vi "Data Displayer.vi"(6 "Fast Controls Only (F)":bool, 7 "Reset":bool, 8 "error in":errorcluster, 10 "All Data":T3 caption="All Data Cluster", 11 "Ref Data Array":T5) -> (0 "error out":errorcluster)   [LabVIEW 2018]
uses:
  Shared Controls/UI Ref Arrays.ctl
  Shared Controls/All Data Cluster.ctl
  Shared Controls/Acq Data.ctl
  Shared Controls/Calculated Data.ctl
  Shared Controls/Post-Analysis Data.ctl
  Gets APU Column Index.vi
panel:
  in  "Post-Analysis Data":T1
  in  "Calculated Values":T2
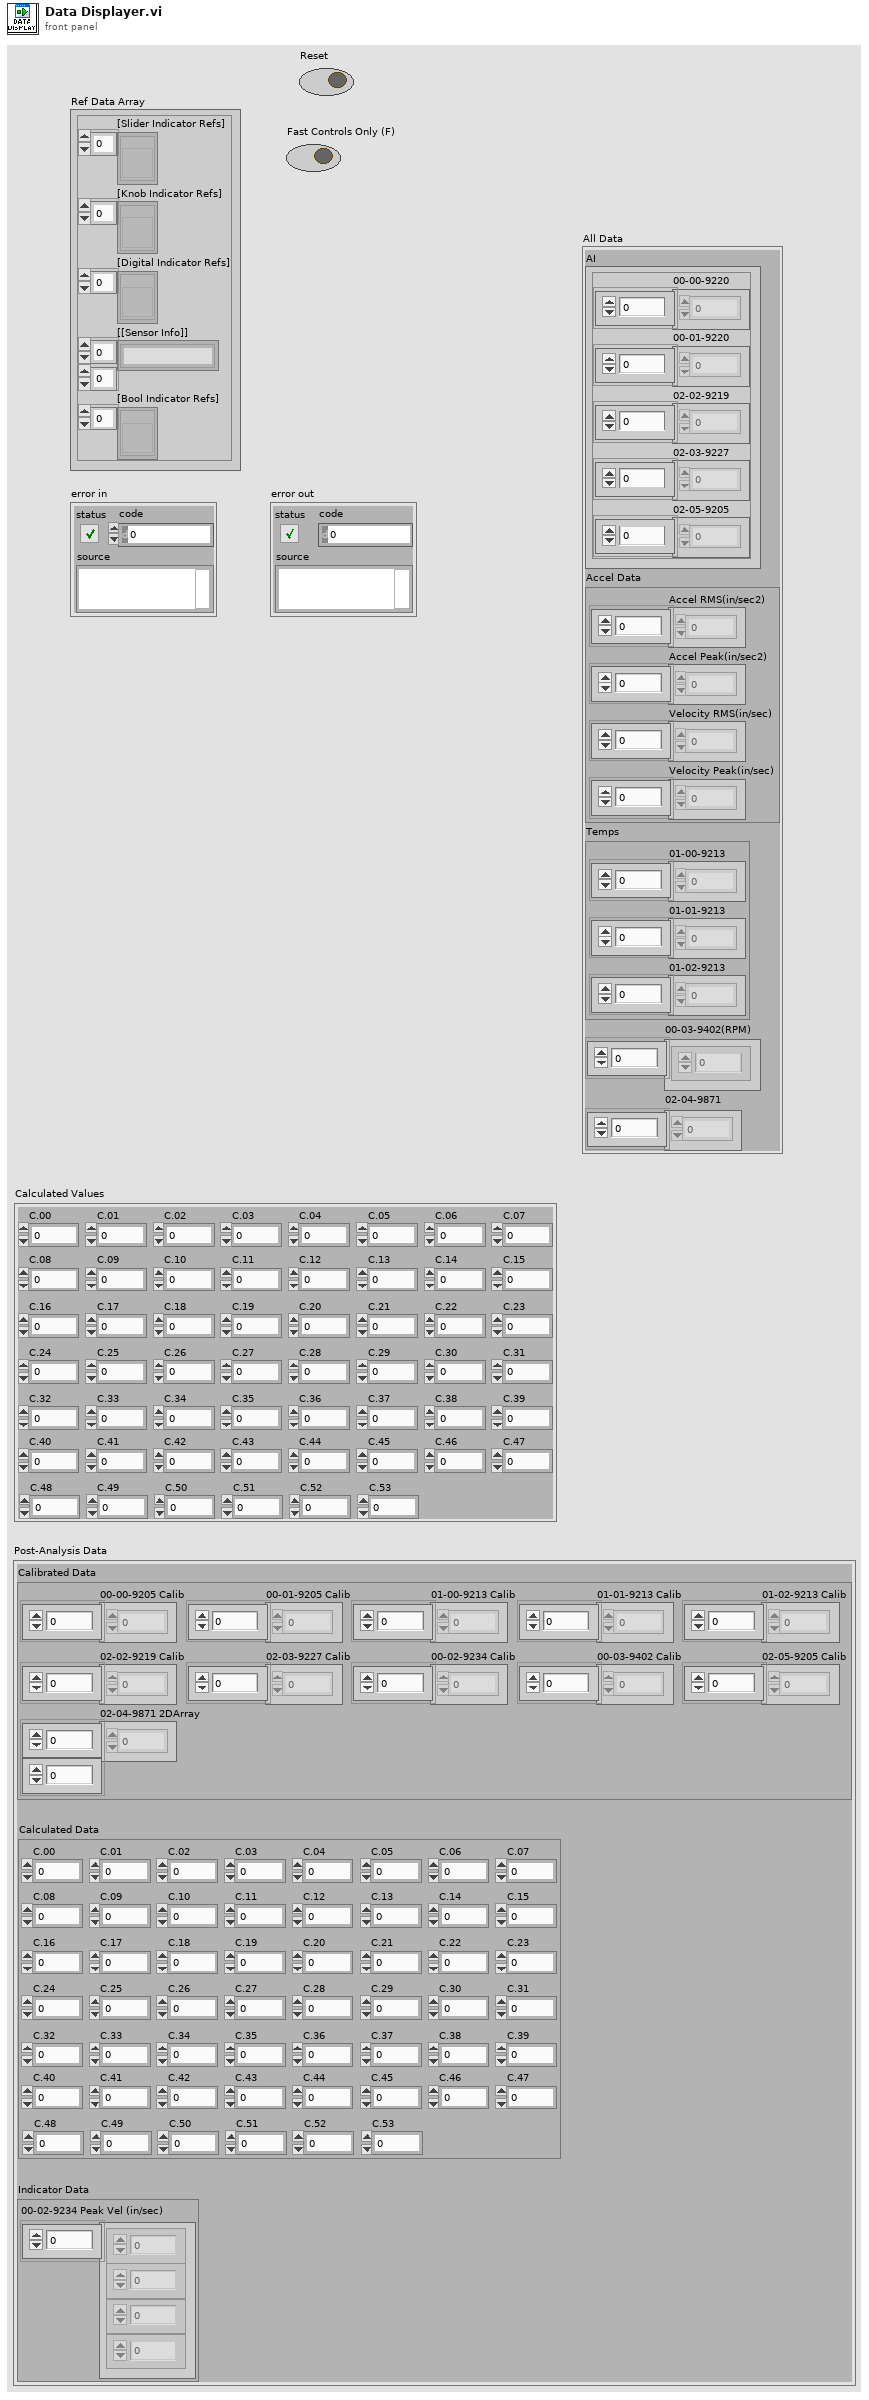
[diagram p1: front panel]
types:
  T1 = typedef "Post-Analysis Data.ctl" = cluster{"Calibrated Data":cluster{"00-00-9205 Calib":dbl[], "00-01-9205 Calib":dbl[], "01-00-9213 Calib":dbl[], "01-01-9213 Calib":dbl[], "01-02-9213 Calib":dbl[], "02-02-9219 Calib":dbl[], "02-03-9227 Calib":dbl[], "00-02-9234 Calib":dbl[], "00-03-9402 Calib":dbl[], "02-05-9205 Calib":dbl[], "02-04-9871 2DArray":dbl[][]}, "Calculated Data":T2, "Indicator Data":cluster{"00-02-9234 Peak Vel (in/sec)":dbl[]}}
  T2 = typedef "Calculated Data.ctl" = cluster{"C.00":dbl, "C.01":dbl, "C.02":dbl, "C.03":dbl, "C.04":dbl, "C.05":dbl, "C.06":dbl, "C.07":dbl, "C.08":dbl, "C.09":dbl, "C.10":dbl, "C.11":dbl, "C.12":dbl, "C.13":dbl, "C.14":dbl, "C.15":dbl, "C.16":dbl, "C.17":dbl, "C.18":dbl, "C.19":dbl, "C.20":dbl, "C.21":dbl, "C.22":dbl, "C.23":dbl, "C.24":dbl, "C.25":dbl, "C.26":dbl, "C.27":dbl, "C.28":dbl, "C.29":dbl, "C.30":dbl, "C.31":dbl, "C.32":dbl, "C.33":dbl, "C.34":dbl, "C.35":dbl, "C.36":dbl, "C.37":dbl, "C.38":dbl, "C.39":dbl, "C.40":dbl, "C.41":dbl, "C.42":dbl, "C.43":dbl, "C.44":dbl, "C.45":dbl, "C.46":dbl, "C.47":dbl, "C.48":dbl, "C.49":dbl, "C.50":dbl, "C.51":dbl, "C.52":dbl, "C.53":dbl}
  T3 = typedef "All Data Cluster.ctl" = cluster{"AI":T4, "Accel Data":cluster{"Accel RMS(in/sec2)":dbl[], "Accel Peak(in/sec2)":dbl[], "Velocity RMS(in/sec)":dbl[], "Velocity Peak(in/sec)":dbl[]}, "Temps":cluster{"01-00-9213":dbl[], "01-01-9213":dbl[], "01-02-9213":dbl[]}, "00-03-9402(RPM)":dbl[], "02-04-9871":dbl[]}
  T4 = typedef "Acq Data.ctl" = cluster{"00-00-9220":dbl[], "00-01-9220":dbl[], "02-02-9219":dbl[], "02-03-9227":dbl[], "02-05-9205":dbl[]}
  T5 = typedef "UI Ref Arrays.ctl" = cluster{"[Slider Indicator Refs]":refnum<vi>[], "[Knob Indicator Refs]":refnum<vi>[], "[Digital Indicator Refs]":refnum<vi>[], "[[Sensor Info]]":string[][], "[Bool Indicator Refs]":refnum<vi>[]}
  T6 = cluster{"Thresold Array":dbl[], "Label Text":string, "Ref type":enum16{"Not Found", "Knob", "Numeric", "Slide", "String", "Boolean"}, "BG Color":u32}
  T7 = typedef "Parsed Tag Cluster.ctl" = cluster{"Whole Tag":string, "# of Sections":u8, "Chassis":u8, "Slot":u8, "Module":string, "Channel":u8, "SubChannel":u8}
  T8 = cluster{"Thresold Array":dbl[], "Label Text":string, "Ref type":enum16{"Not Found", "Knob", "Numeric", "Slide", "String", "Boolean"}, "BG Color":u32}[]
  T9 = enum16{"Not Found", "Knob", "Numeric", "Slide", "String", "Boolean"}
  T10 = cluster{"Thresold Array":dbl[], "Label.Text":string, "Ref type":enum16{"Not Found", "Knob", "Numeric", "Slide", "String", "Boolean"}, "BG Color":u32}
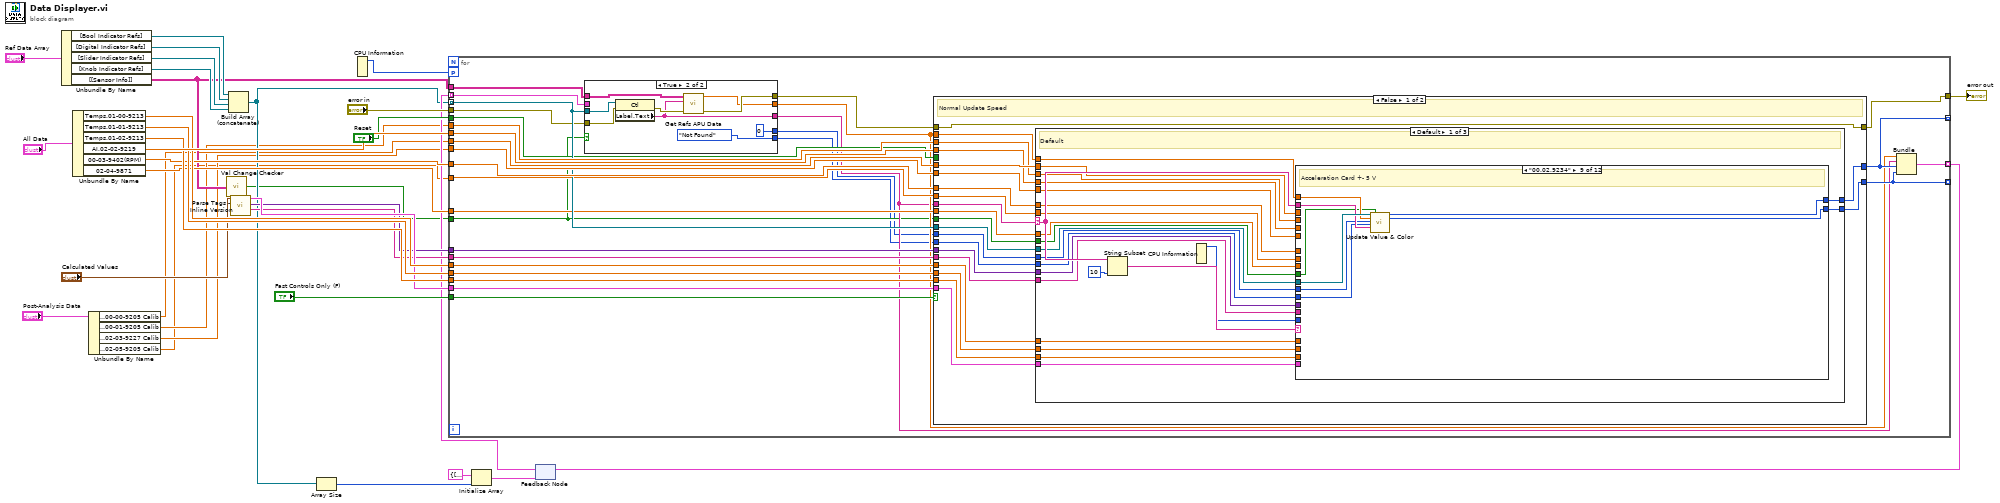
[diagram p0: block diagram]
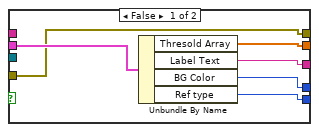
[diagram p2: hidden frame]
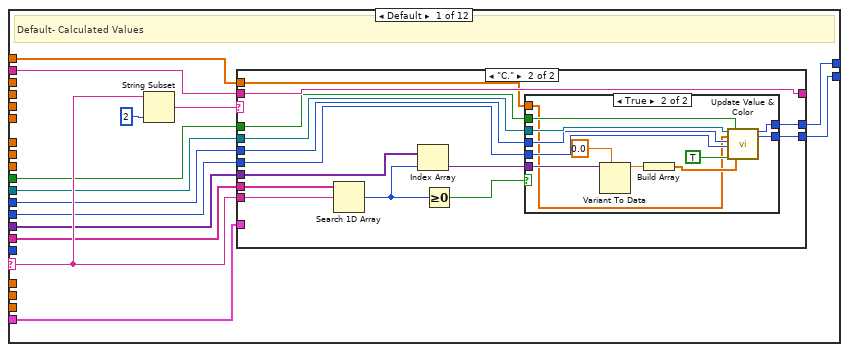
[diagram p3: hidden frame]
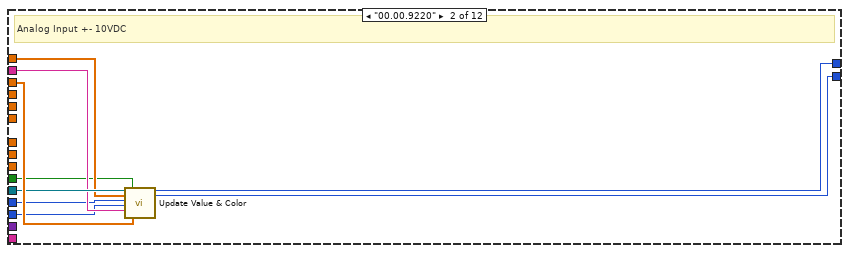
[diagram p6: hidden frame]
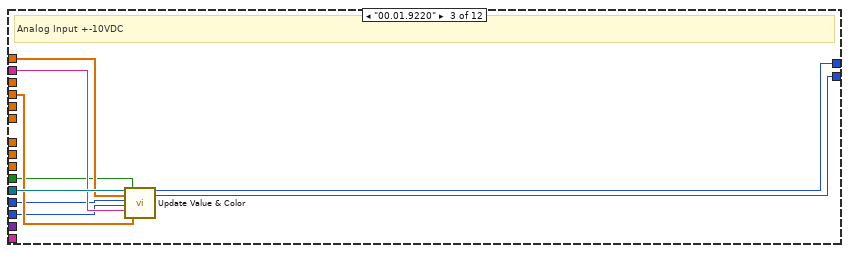
[diagram p7: hidden frame]
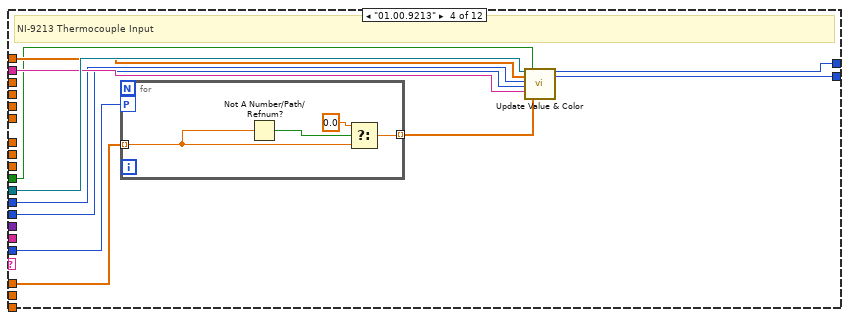
[diagram p8: hidden frame]
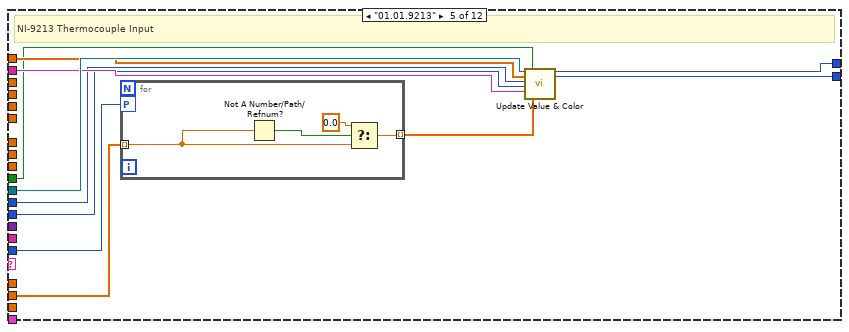
[diagram p9: hidden frame]
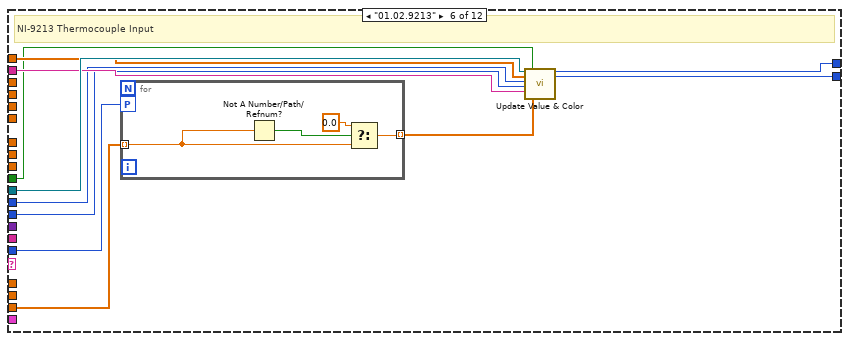
[diagram p10: hidden frame]
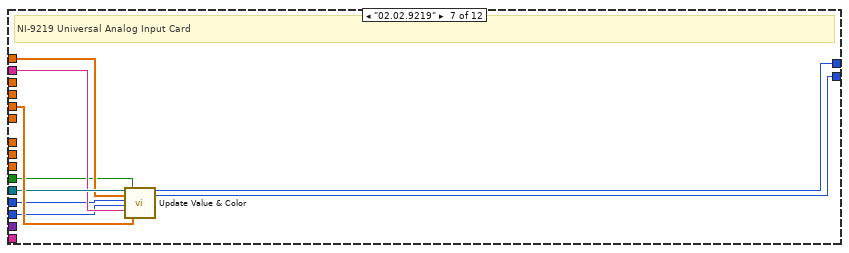
[diagram p11: hidden frame]
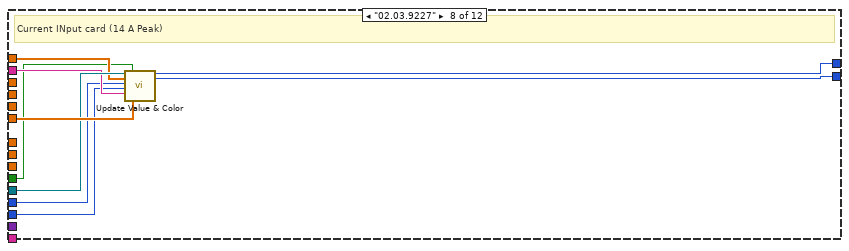
[diagram p12: hidden frame]
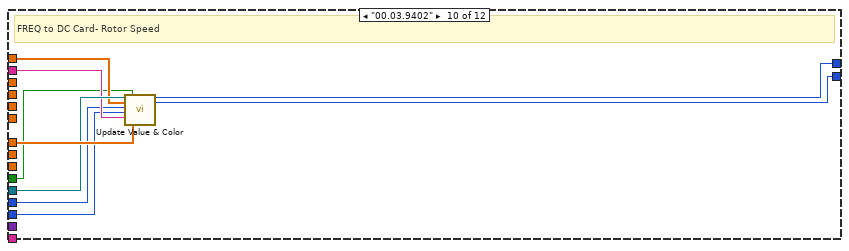
[diagram p13: hidden frame]
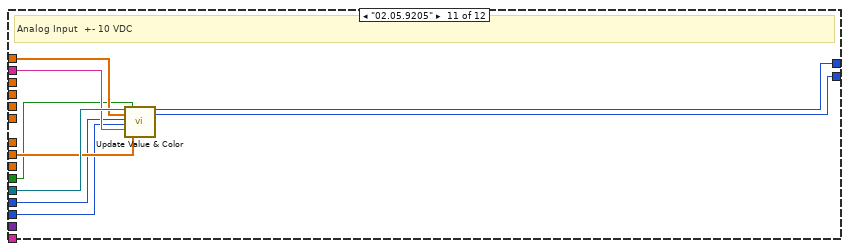
[diagram p14: hidden frame]
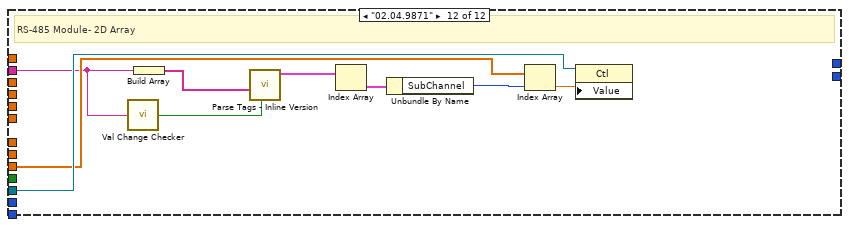
[diagram p15: hidden frame]
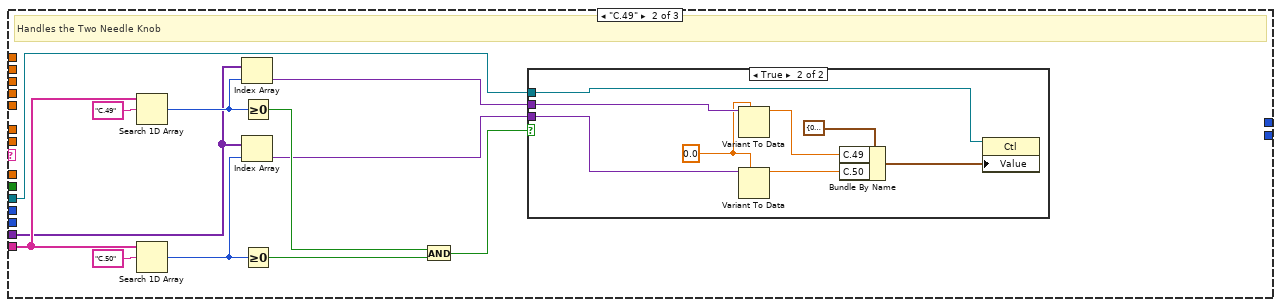
[diagram p16: hidden frame]
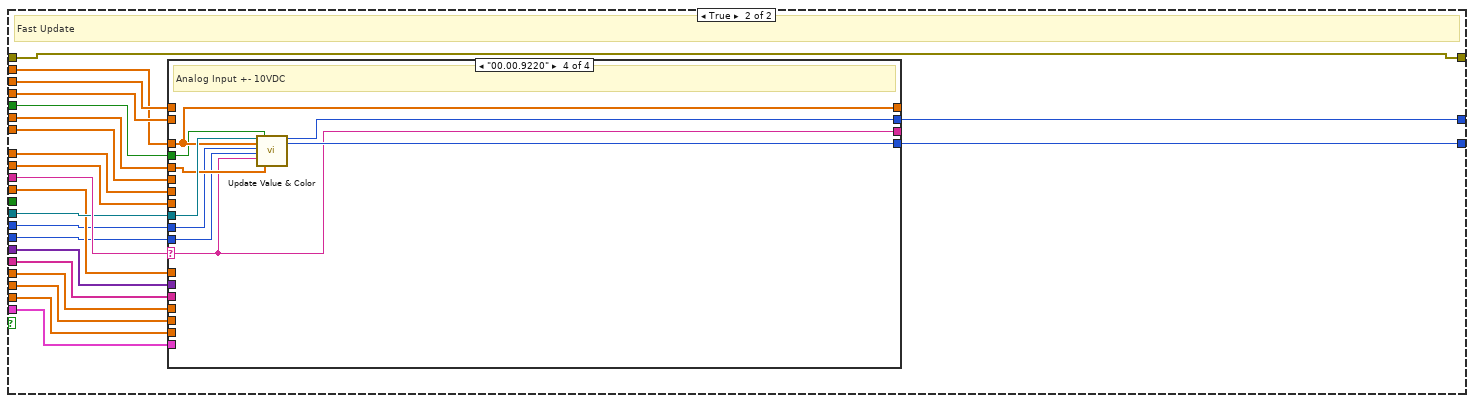
[diagram p19: hidden frame]
diagram:
  n1 = Unbundle By Name("Ref Data Array") -> ("[Bool Indicator Refs]"=w33:refnum<vi>[], "[Digital Indicator Refs]"=w34:refnum<vi>[], "[Slider Indicator Refs]"=w31:refnum<vi>[], "[Knob Indicator Refs]"=w32:refnum<vi>[], "[[Sensor Info]]"=w10:string[][])
  n2 = Unbundle By Name("All Data") -> ("Temps.01-00-9213"=w24:dbl[], "Temps.01-01-9213"=w29:dbl[], "Temps.01-02-9213"=w28:dbl[], "AI.02-02-9219"=w30:dbl[], "00-03-9402(RPM)"=w17:dbl[], "02-04-9871"=w21:dbl[])
  n3 = Unbundle By Name("Post-Analysis Data") -> ("Calibrated Data.00-00-9205 Calib"=w4:dbl[], "Calibrated Data.00-01-9205 Calib"=w3:dbl[], "Calibrated Data.02-03-9227 Calib"=w2:dbl[], "Calibrated Data.02-05-9205 Calib"=w1:dbl[])
  n4 = call "Val Change Checker.vi"("Current Value in"=w10) -> ("Value Change?"=w9:bool)
  n5 = Build Array (concatenate)(w33, w34, w31, w32) -> (w15:refnum<vi>[])
  n6 = call "Parse Tags - Inline Version.vi"("Cluster of Controls"="Calculated Values") -> ("[Whole Tags]"=w19:string[], "[VData out]"=w22:variant[], "[Parsed Tags]"=w23:T7[])  [unwired: 7 in, 1 out]
  n7 = Array Size(array=w15) -> (size(s)=w14:i32)
  n8 = CPU Information() -> (4:w8:i32)  [unwired: 3 out]
  n9 = Initialize Array(T6 {"Thresold Array"=[], "Label Text"="", "Ref type"=enum."Not Found", "BG Color"=0} ("output cluster"), w14) -> (w12:T8)
  n10 = feedback #1(w12) -> (w16:T8)
  n11 = for {
    tunnel: w4 -> [w63]
    tunnel: w3 -> [w62]
    tunnel: w24 -> [w61]
    tunnel: w29 -> [w60]
    tunnel: w28 -> [w59]
    tunnel: w17 -> [w58]
    tunnel: w30 -> [w57]
    tunnel: w2 -> [w56]
    tunnel: "error in" -> [w46]
    tunnel: [w44] -> w25
    tunnel: w10 -> [w55]
    tunnel: w15 -> [w54] mode=indexing
    tunnel: w1 -> [w53]
    tunnel: w23 -> [w52]
    tunnel: w22 -> [w51]
    tunnel: w21 -> [w50]
    tunnel: "Fast Controls Only (F)" -> [w49]
    tunnel: w19 -> [w48]
    tunnel: "Reset" -> [w47]
    workers-P: w8 -> [_]
    tunnel: [w43] -> _ mode=indexing
    tunnel: [w42] -> _ mode=indexing
    tunnel: [w41] -> w11 mode=indexing
    tunnel: w16 -> [w38] mode=indexing
    tunnel: w9 -> [w37]
    n12 = case shown="True" w37 {
      tunnel: w55 -> [_ w77]
      tunnel: w54 -> [_ w76]
      tunnel: w46 -> [w66 w75]
      tunnel: [w66 w74] -> w45
      tunnel: [w68 w73] -> w40
      tunnel: [w67 w72] -> w39
      tunnel: w38 -> [w69 _]
      tunnel: [w65 u32 0 ("BG Color")] -> w36
      tunnel: [w64 T9."Not Found" ("Ref type")] -> w35
      frame False {
        n13 = Unbundle By Name(w69) -> ("Thresold Array"=w68:dbl[], "Label Text"=w67:string, "BG Color"=w65:u32, "Ref type"=w64:T9)
      }
      frame True {
        n14 = property class="Ctl"(reference=w76, error in=w75) -> (error out=w78:errorcluster, "Label.Text"=w72:string)  [unwired: 1 out]
        n15 = call "Get Refs APU Data.vi"("error in (no error)"=w78, "Label.Text"=w72, "APU Setup"=w77) -> ("error out"=w74:errorcluster, "Thresold Array"=w73:dbl[])  [unwired: 7 in]
      }
    }
    n16 = case shown="False" w49 {
      tunnel: w63 -> [w100 w323]
      tunnel: w62 -> [w99 w322]
      tunnel: w61 -> [w98 w321]
      tunnel: w60 -> [w97 w320]
      tunnel: w59 -> [w96 w319]
      tunnel: w58 -> [w95 w318]
      tunnel: w57 -> [w94 w317]
      tunnel: w56 -> [w93 w316]
      tunnel: w39 -> [w92 w315]
      tunnel: w40 -> [w91 w314]
      tunnel: w54 -> [w90 w313]
      tunnel: w53 -> [w89 w312]
      tunnel: w52 -> [w88 w311]
      tunnel: w51 -> [w87 w310]
      tunnel: w50 -> [w86 w309]
      tunnel: w48 -> [w85 w308]
      tunnel: w47 -> [_ w307]
      tunnel: [w84 w306] -> w44
      tunnel: w45 -> [w84 w306]
      tunnel: [w83 w304] -> w43
      tunnel: [w82 w305] -> w42
      tunnel: w37 -> [w81 _]
      tunnel: w36 -> [w80 w303]
      tunnel: w35 -> [w79 w302]
      frame False {
        # "Normal Update Speed"
        n17 = case shown="Default" w92 {
          selector: w92 -> [w122 _ _]
          tunnel: w100 -> [w101 _ _]
          tunnel: w99 -> [w121 _ _]
          tunnel: w98 -> [w120 _ _]
          tunnel: w97 -> [w119 _ _]
          tunnel: w96 -> [w118 _ _]
          tunnel: w95 -> [w115 _ _]
          tunnel: w94 -> [w117 _ _]
          tunnel: w93 -> [w116 _ _]
          tunnel: w91 -> [w102 _ _]
          tunnel: w90 -> [w114 w293 _]
          tunnel: w89 -> [w113 _ _]
          tunnel: w88 -> [w112 _ _]
          tunnel: w87 -> [w111 w284 _]
          tunnel: w86 -> [w110 _ _]
          tunnel: w85 -> [w109 w285 _]
          tunnel: [w107 _ _] -> w83
          tunnel: [w106 _ _] -> w82
          tunnel: w81 -> [w105 _ _]
          tunnel: w80 -> [w104 _ _]
          tunnel: w79 -> [w103 _ _]
          frame Default {
            # "Default"
            n18 = String Subset(string=w122, length (rest)=10 ("length (rest)")) -> (substring=w123:string)  [unwired: 1 in]
            n19 = CPU Information() -> (4:w108:i32)  [unwired: 3 out]
            n20 = case shown="\"00.02.9234\"" w123 {
              selector: w123 -> [w137 _ _ _ _ _ _ _ _ _ _ _]
              tunnel: w122 -> [w129 w169 w179 w187 w202 w217 w232 w241 w251 w258 w267 w274]
              tunnel: w101 -> [_ w174 _ _ _ _ _ _ _ _ _ _]
              tunnel: w121 -> [_ _ w182 _ _ _ _ _ _ _ _ _]
              tunnel: w120 -> [_ _ _ w193 _ _ _ _ _ _ _ _]
              tunnel: w119 -> [_ _ _ _ w207 _ _ _ _ _ _ _]
              tunnel: w118 -> [_ _ _ _ _ w222 _ _ _ _ _ _]
              tunnel: w117 -> [_ _ _ _ _ _ w237 _ _ _ _ _]
              tunnel: w116 -> [_ _ _ _ _ _ _ w246 _ _ _ _]
              tunnel: w115 -> [_ _ _ _ _ _ _ _ _ w263 _ _]
              tunnel: w102 -> [w125 w170 w178 w188 w203 w218 w233 w242 w250 w259 w268 _]
              tunnel: w114 -> [w135 w173 w183 w194 w209 w224 w236 w245 w254 w262 w272 w280]
              tunnel: w113 -> [_ _ _ _ _ _ _ _ _ _ w271 _]
              tunnel: w112 -> [w134 _ _ _ _ _ _ _ _ _ _ _]
              tunnel: w111 -> [w133 _ _ _ _ _ _ _ _ _ _ _]
              tunnel: w110 -> [_ _ _ _ _ _ _ _ _ _ _ w276]
              tunnel: w109 -> [w132 _ _ _ _ _ _ _ _ _ _ _]
              tunnel: w108 -> [_ _ _ w191 w206 w221 _ _ _ _ _ _]
              tunnel: [w130 w171 w180 w190 w204 w219 w234 w243 w252 w260 w269 _] -> w107
              tunnel: [w131 w172 w181 w189 w205 w220 w235 w244 w253 w261 w270 _] -> w106
              tunnel: w105 -> [w128 w168 w177 w186 w201 w216 w231 w240 w247 w257 w264 _]
              tunnel: w104 -> [w127 w167 w176 w185 w200 w215 w230 w239 w249 w256 w266 _]
              tunnel: w103 -> [w126 w166 w175 w184 w199 w214 w229 w238 w248 w255 w265 _]
              frame Default {
                # "Default- Calculated Values"
                n21 = String Subset(string=w137, length (rest)=2 ("length (rest)")) -> (substring=w138:string)  [unwired: 1 in]
                n22 = case shown="\"C.\"" w138 {
                  tunnel: w137 -> [_ w152]
                  tunnel: w135 -> [_ w149]
                  tunnel: w134 -> [_ _]
                  tunnel: w133 -> [_ w151]
                  tunnel: w132 -> [_ w153]
                  tunnel: [_ w146] -> w131
                  tunnel: [_ w145] -> w130
                  tunnel: [w139 w144] -> _
                  tunnel: w129 -> [w139 w144]
                  tunnel: w128 -> [_ w143]
                  tunnel: w127 -> [_ w142]
                  tunnel: w126 -> [_ w141]
                  tunnel: w125 -> [_ w140]
                  frame Default {
                  }
                  frame "C." {
                    n23 = Search 1D Array(1D array=w153, element=w152) -> (index of element=w150:i32)  [unwired: 1 in]
                    n24 = Index Array(array=w151, index=w150) -> (element=w148:variant)
                    n25 = Greater Or Equal To 0?(x=w150) -> (x >= 0?=w147:bool)
                    n26 = case shown="True" w147 {
                      tunnel: w149 -> [_ w165]
                      tunnel: w148 -> [_ w163]
                      tunnel: [_ w159] -> w146
                      tunnel: [_ w158] -> w145
                      tunnel: w143 -> [_ w157]
                      tunnel: w142 -> [_ w156]
                      tunnel: w141 -> [_ w155]
                      tunnel: w140 -> [_ w154]
                      frame False {
                      }
                      frame True {
                        n27 = Variant To Data(type=0.0 ("x"), Variant=w163) -> (data=w161:dbl)  [unwired: 1 in, 1 out]
                        n28 = Build Array(w161) -> (w160:dbl[])
                        n29 = call "Update Value & Color.vi"("Ref In"=w165, "Thresold Array & Range Max"=w154, "BG Color In"=w156, "Ref type In"=w155, "Calculated Value (F)?"=TRUE, "Val Change?"=w157, "Value In"=w160) -> ("Ref type"=w159:T9, "BG Color"=w158:u32)  [unwired: 11 in]
                      }
                    }
                  }
                }
              }
              frame "00.00.9220" {
                # "Analog Input +- 10VDC"
                n30 = call "Update Value & Color.vi"("Ref In"=w173, "Thresold Array & Range Max"=w170, "BG Color In"=w167, "Ref type In"=w166, "Control Label In"=w169, "Val Change?"=w168, "Value In"=w174) -> ("Ref type"=w172:T9, "BG Color"=w171:u32)  [unwired: 11 in]
              }
              frame "00.01.9220" {
                # "Analog Input +-10VDC"
                n31 = call "Update Value & Color.vi"("Ref In"=w183, "Thresold Array & Range Max"=w178, "BG Color In"=w176, "Ref type In"=w175, "Control Label In"=w179, "Val Change?"=w177, "Value In"=w182) -> ("Ref type"=w181:T9, "BG Color"=w180:u32)  [unwired: 11 in]
              }
              frame "01.00.9213" {
                # "NI-9213 Thermocouple Input"
                n32 = for {
                  tunnel: w193 -> [w197] mode=indexing
                  tunnel: [w195] -> w192 mode=indexing
                  workers-P: w191 -> [_]
                  n33 = Not A Number/Path/Refnum?(number/path/refnum=w197) -> (NaN/Path/Refnum?=w198:bool)
                  n34 = Select(t=0.0, s=w198, f=w197) -> (s? t:f=w195:dbl)
                }
                n35 = call "Update Value & Color.vi"("Ref In"=w194, "Thresold Array & Range Max"=w188, "BG Color In"=w185, "Ref type In"=w184, "Control Label In"=w187, "Val Change?"=w186, "Value In"=w192) -> ("Ref type"=w189:T9, "BG Color"=w190:u32)  [unwired: 11 in]
              }
              frame "01.01.9213" {
                # "NI-9213 Thermocouple Input"
                n36 = for {
                  tunnel: w207 -> [w212] mode=indexing
                  tunnel: [w210] -> w208 mode=indexing
                  workers-P: w206 -> [_]
                  n37 = Not A Number/Path/Refnum?(number/path/refnum=w212) -> (NaN/Path/Refnum?=w213:bool)
                  n38 = Select(t=0.0, s=w213, f=w212) -> (s? t:f=w210:dbl)
                }
                n39 = call "Update Value & Color.vi"("Ref In"=w209, "Thresold Array & Range Max"=w203, "BG Color In"=w200, "Ref type In"=w199, "Control Label In"=w202, "Val Change?"=w201, "Value In"=w208) -> ("Ref type"=w205:T9, "BG Color"=w204:u32)  [unwired: 11 in]
              }
              frame "01.02.9213" {
                # "NI-9213 Thermocouple Input"
                n40 = for {
                  tunnel: w222 -> [w227] mode=indexing
                  tunnel: [w225] -> w223 mode=indexing
                  workers-P: w221 -> [_]
                  n41 = Not A Number/Path/Refnum?(number/path/refnum=w227) -> (NaN/Path/Refnum?=w228:bool)
                  n42 = Select(t=0.0, s=w228, f=w227) -> (s? t:f=w225:dbl)
                }
                n43 = call "Update Value & Color.vi"("Ref In"=w224, "Thresold Array & Range Max"=w218, "BG Color In"=w215, "Ref type In"=w214, "Control Label In"=w217, "Val Change?"=w216, "Value In"=w223) -> ("Ref type"=w220:T9, "BG Color"=w219:u32)  [unwired: 11 in]
              }
              frame "02.02.9219" {
                # "NI-9219 Universal Analog Input Card"
                n44 = call "Update Value & Color.vi"("Ref In"=w236, "Thresold Array & Range Max"=w233, "BG Color In"=w230, "Ref type In"=w229, "Control Label In"=w232, "Val Change?"=w231, "Value In"=w237) -> ("Ref type"=w235:T9, "BG Color"=w234:u32)  [unwired: 11 in]
              }
              frame "02.03.9227" {
                # "Current INput card (14 A Peak)"
                n45 = call "Update Value & Color.vi"("Ref In"=w245, "Thresold Array & Range Max"=w242, "BG Color In"=w239, "Ref type In"=w238, "Control Label In"=w241, "Val Change?"=w240, "Value In"=w246) -> ("Ref type"=w244:T9, "BG Color"=w243:u32)  [unwired: 11 in]
              }
              frame "00.02.9234" {
                # "Acceleration Card +- 5 V"
                n46 = call "Update Value & Color.vi"("Ref In"=w254, "Thresold Array & Range Max"=w250, "BG Color In"=w249, "Ref type In"=w248, "Control Label In"=w251, "Val Change?"=w247) -> ("Ref type"=w253:T9, "BG Color"=w252:u32)  [unwired: 12 in]
              }
              frame "00.03.9402" {
                # "FREQ to DC Card- Rotor Speed"
                n47 = call "Update Value & Color.vi"("Ref In"=w262, "Thresold Array & Range Max"=w259, "BG Color In"=w256, "Ref type In"=w255, "Control Label In"=w258, "Val Change?"=w257, "Value In"=w263) -> ("Ref type"=w261:T9, "BG Color"=w260:u32)  [unwired: 11 in]
              }
              frame "02.05.9205" {
                # "Analog Input  +- 10 VDC"
                n48 = call "Update Value & Color.vi"("Ref In"=w272, "Thresold Array & Range Max"=w268, "BG Color In"=w266, "Ref type In"=w265, "Control Label In"=w267, "Val Change?"=w264, "Value In"=w271) -> ("Ref type"=w270:T9, "BG Color"=w269:u32)  [unwired: 11 in]
              }
              frame "02.04.9871" {
                # "RS-485 Module- 2D Array"
                n49 = call "Val Change Checker.vi"("Current Value in"=w274) -> ("Value Change?"=w275:bool)
                n50 = Build Array(w274) -> (w279:string[])
                n51 = call "Parse Tags - Inline Version.vi"("New Tag Info (F)"=w275, "[Tags]"=w279) -> ("[Parsed Tags]"=w278:T7[])  [unwired: 6 in, 3 out]
                n52 = Index Array(array=w278) -> (element=w277:T7)  [unwired: 1 in]
                n53 = Unbundle By Name(w277) -> ("SubChannel"=w273:u8)
                n54 = Index Array(array=w276, index=w273) -> (element=w281:dbl)
                n55 = property class="Ctl"(reference=w280, "Value"=w281) -> ()  [unwired: 1 in, 2 out]
              }
            }
          }
          frame "C.49" {
            # "Handles the Two Needle Knob"
            n56 = Search 1D Array(1D array=w285, element="C.49") -> (index of element=w291:i32)  [unwired: 1 in]
            n57 = Search 1D Array(1D array=w285, element="C.50") -> (index of element=w287:i32)  [unwired: 1 in]
            n58 = Index Array(array=w284, index=w291) -> (element=w289:variant)
            n59 = Index Array(array=w284, index=w287) -> (element=w283:variant)
            n60 = Greater Or Equal To 0?(x=w291) -> (x >= 0?=w288:bool)
            n61 = Greater Or Equal To 0?(x=w287) -> (x >= 0?=w282:bool)
            n62 = And(x=w288, y=w282) -> (x .and. y?=w292:bool)
            n63 = case shown="True" w292 {
              tunnel: w293 -> [_ w301]
              tunnel: w289 -> [_ w298]
              tunnel: w283 -> [_ w295]
              frame False {
              }
              frame True {
                w296 = 0.0 ("C.26")
                n64 = Variant To Data(type=w296, Variant=w298) -> (data=w297:dbl)  [unwired: 1 in, 1 out]
                n65 = Variant To Data(type=w296, Variant=w295) -> (data=w294:dbl)  [unwired: 1 in, 1 out]
                n66 = Bundle By Name(cluster=cluster{"C.49":dbl, "C.50":dbl} {"C.49"=0.0, "C.50"=0.0} ("Value"), "C.49"=w297, "C.50"=w294) -> (w300:cluster{"C.49":dbl, "C.50":dbl})
                n67 = property class="Ctl"(reference=w301, "Value"=w300) -> ()  [unwired: 1 in, 2 out]
              }
            }
          }
          frame "00.03.9402", "02.05.9205.01", "02.05.9205.01 Max" {
            # "Used in Fast Update Case"
          }
        }
      }
      frame True {
        # "Fast Update"
        n68 = case shown="\"00.00.9220\"" w315 {
          selector: w315 -> [w324 w326 w342 w356]
          tunnel: w323 -> [_ _ _ w360]
          tunnel: w322 -> [_ _ _ _]
          tunnel: w321 -> [_ _ _ _]
          tunnel: w320 -> [_ _ _ _]
          tunnel: w319 -> [_ _ _ _]
          tunnel: w318 -> [_ _ w347 _]
          tunnel: w317 -> [_ _ _ _]
          tunnel: w316 -> [_ _ w346 _]
          tunnel: w314 -> [w325 w327 w343 w357]
          tunnel: w313 -> [_ w329 w348 w361]
          tunnel: w312 -> [_ w334 _ _]
          tunnel: w311 -> [_ _ _ _]
          tunnel: w310 -> [_ _ _ _]
          tunnel: w309 -> [_ _ _ _]
          tunnel: w308 -> [_ _ _ _]
          tunnel: w307 -> [_ w333 _ w355]
          tunnel: [_ _ _ w359] -> w305
          tunnel: [_ _ _ w358] -> w304
          tunnel: [w325 w327 w343 w357] -> _
          tunnel: [w324 w326 w342 w356] -> _
          tunnel: w303 -> [_ _ _ w354]
          tunnel: w302 -> [_ _ _ w353]
          frame Default {
            # "Default"
          }
          frame "02.05.9205.01", "02.05.9205.01 Max" {
            # "Starter Current Reading, Find Max Value"
            n69 = property class="Ctl"(reference=w329) -> (reference out=w328:refnum<vi>, "Value"=w332:variant)  [unwired: 1 in, 1 out]
            n70 = Index Array(array=w334, index=1) -> (element=w330:dbl)
            n71 = Variant To Data(type=w330, Variant=w332) -> (data=w331:dbl)  [unwired: 1 in, 1 out]
            n72 = Select(t=0.0, s=w333, f=w331) -> (s? t:f=w338:dbl)
            n73 = Equal?(x=w326, y="02.05.9205.01") -> (x = y?=w335:bool)
            n74 = Max & Min(x=w330, y=w338) -> (max(x,y)=w340:dbl)  [unwired: 1 out]
            n75 = Select(t=w330, s=w335, f=w340) -> (s? t:f=w337:dbl)
            n76 = property class="Ctl"(reference=w328, "Value"=w337) -> ()  [unwired: 1 in, 2 out]
          }
          frame "00.03.9402" {
            # "N1 and N2 Rotor Speed 00.03.9402.00 and 02.03.9227.01"
            n77 = Index Array(array=w346, index=1) -> (element=w344:dbl)
            n78 = Index Array(array=w347, index=0) -> (element=w351:dbl)
            n79 = Bundle By Name(cluster=cluster{"N1":dbl, "N2":dbl} {"N1"=0.0, "N2"=0.0} ("Value"), "N1"=w351, "N2"=w344) -> (w352:cluster{"N1":dbl, "N2":dbl})
            n80 = property class="Ctl"(reference=w348, "Value"=w352) -> ()  [unwired: 1 in, 2 out]
          }
          frame "00.00.9220" {
            # "Analog Input +- 10VDC"
            n81 = call "Update Value & Color.vi"("Ref In"=w361, "Thresold Array & Range Max"=w357, "BG Color In"=w354, "Ref type In"=w353, "Control Label In"=w356, "Val Change?"=w355, "Value In"=w360) -> ("Ref type"=w359:T9, "BG Color"=w358:u32)  [unwired: 11 in]
          }
        }
      }
    }
    n82 = Bundle("Thresold Array"=w40, "Label.Text"=w39, "Ref type"=w42, "BG Color"=w43) -> (w41:T10)  [unwired: 1 in]
  }
  "error out" <- w25
  n83 = feedback-in #1(w11) -> ()
